vi "toml_api_serialize.vi"(8 "error in (no error)":errorcluster, 11 "sections":T1(array[cluster])) -> (0 "error out":errorcluster, 3 "text out":string)   [LabVIEW 2017]
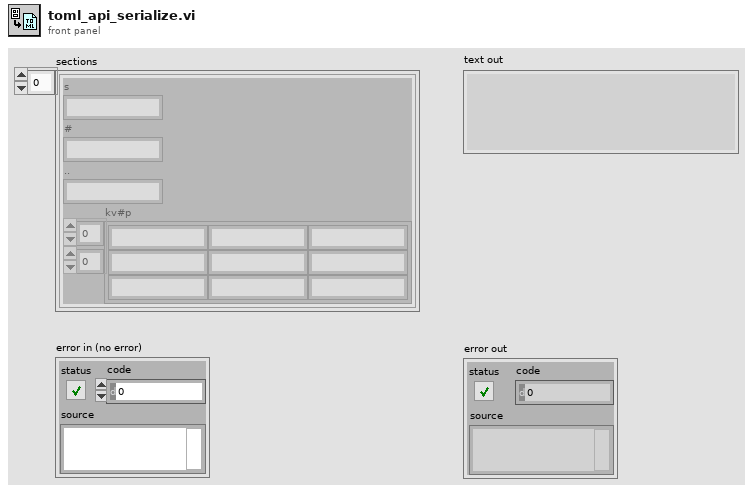
[diagram p1: front panel]
types:
  T1 = cluster{"s":string, "#":string, "..":string, "kv#p":string[][]}[]
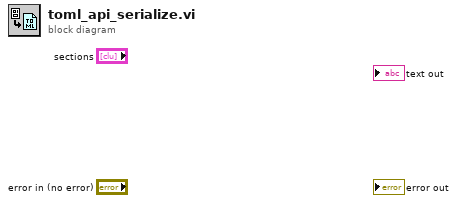
[diagram p0: block diagram]
diagram:
